vi "Ping Sensor.vi"(8 "error in":errorcluster, 11 "VisionServerRef in":T1) -> (0 "error out":errorcluster, 3 "VisionServerRef out":T1)   [LabVIEW 2016, in "Vision Server.lvclass"]
uses:
  Vision Server.lvclass
  typedef/Vision Server Ref.ctl
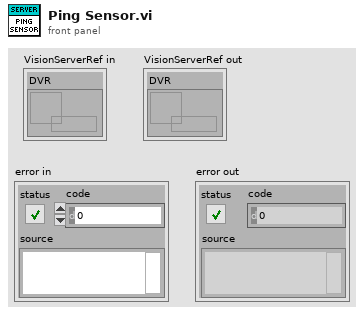
[diagram p1: front panel]
types:
  T1 = typedef "Vision Server.lvclass/Vision Server Ref.ctl" = cluster{"DVR":refnum<data-value>}
  T2 = typedef "Vision Server.lvclass/Message Type.ctl" = cluster{"type":string, "message":string}
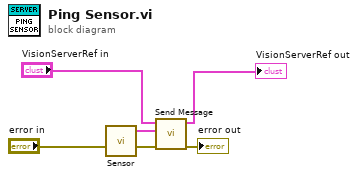
[diagram p0: block diagram]
diagram:
  n1 = call "Sensor.vi"() -> ("camera mode vision"=w3:T2)  [unwired: 2 in]
  n2 = call "Send Message.vi"("error in"="error in", "Message"=w3, "VisionServerRef in"="VisionServerRef in") -> ("error out"=→"error out":errorcluster, "VisionServerRef out"=→"VisionServerRef out":T1)  [unwired: 7 in]
